vi "Find Header Value - Single.vi"(7 "Header":string, 8 "error in (no error)":errorcluster, 10 "headers":T1[](array[typedef])) -> (0 "error out":errorcluster, 1 "Found?":bool, 2 "Value":string)   [LabVIEW 2020, in "Blue Easy HTTP OpenSource.lvlib"]
doc: "Finds the value of a specific Header from a list of HTTP headers and values.\n\nThe Header input is not case sensitive."
uses:
  Blue Easy HTTP OpenSource.lvlib
  HTTP Header.ctl
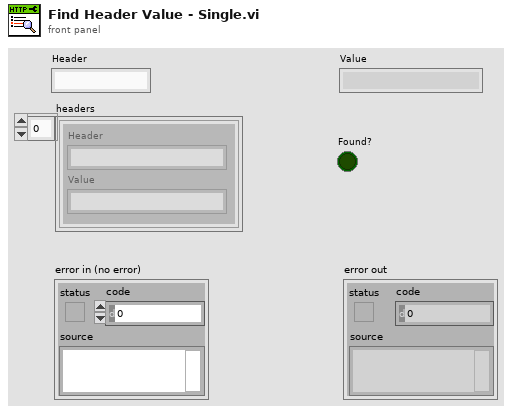
[diagram p1: front panel]
types:
  T1 = typedef "Blue Easy HTTP OpenSource.lvlib/HTTP Header.ctl" = cluster{"Header":string, "Value":string}
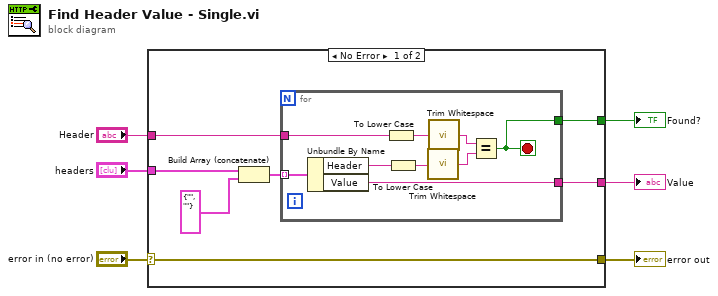
[diagram p0: block diagram]
diagram:
  n1 = case shown="No Error" "error in (no error)" {
    selector: "error in (no error)" -> [w13 w23]
    tunnel: [w13 w23] -> w5
    tunnel: [w10 _] -> w4
    tunnel: [w9 _] -> w3
    tunnel: "headers" -> [w8 _]
    tunnel: "Header" -> [w7 _]
    frame No Error {
      n2 = Build Array (concatenate)(w8, T1 {"Header"="", "Value"=""} ("HTTP Header")) -> (w11:T1[])
      n3 = for {
        tunnel: w11 -> [w18] mode=indexing
        tunnel: [w16] -> w9
        tunnel: [w15] -> w10
        tunnel: w7 -> [w14]
        stop <- w16 stop-if-true
        n4 = Unbundle By Name(w18) -> ("Header"=w17:string, "Value"=w15:string)
        n5 = To Lower Case(string=w14) -> (all lower case string=w21:string)
        n6 = To Lower Case(string=w17) -> (all lower case string=w22:string)
        n7 = call <vilib>:"Trim Whitespace.vi"("string"=w22) -> ("trimmed string"=w19:string)  [unwired: 1 in]
        n8 = call <vilib>:"Trim Whitespace.vi"("string"=w21) -> ("trimmed string"=w20:string)  [unwired: 1 in]
        n9 = Equal?(x=w20, y=w19) -> (x = y?=w16:bool)
      }
    }
    frame Error {
    }
  }
  "error out" <- w5
  "Found?" <- w3
  "Value" <- w4
